vi "SetRemoteControl.vi"(0 "reference in":refnum<class "Button.lvclass">, 7 "RemoteControl":refnum<class "RemoteControl.lvclass">, 11 "Error In":errorcluster) -> (4 "reference out":refnum<class "Button.lvclass">, 15 "Error Out":errorcluster)   [LabVIEW 2024, in "Button.lvclass"]
uses:
  Button.lvclass
  RemoteControl_class/RemoteControl.lvclass
  Button.lvclass/Button.ctl
panel:
  # "Connector Pane"
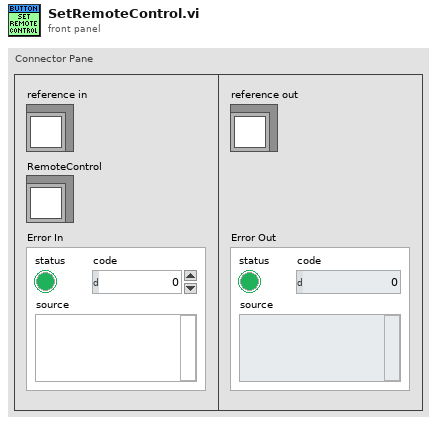
[diagram p1: front panel]
types:
  T1 = typedef "Button.lvclass/ObjectAttributes.ctl" = cluster{"RemoteControl":refnum<class "RemoteControl.lvclass">}
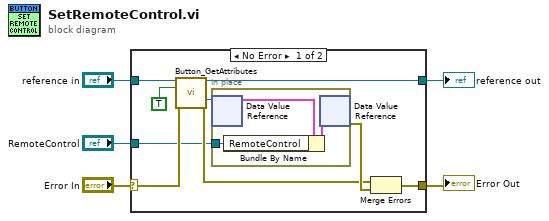
[diagram p0: block diagram]
diagram:
  n1 = case shown="No Error" "Error In" {
    selector: "Error In" -> [w12 w19]
    tunnel: [w7 w19] -> w4
    tunnel: [w13 w18] -> w2
    tunnel: "reference in" -> [w14 w18]
    tunnel: "RemoteControl" -> [w6 _]
    frame No Error {
      n2 = call "Button_GetAttributes.vi"("reference in"=w14, "OnlyGetDvrReference(False)"=TRUE, "Error In"=w12) -> ("reference out"=w13:refnum<class "Button.lvclass">, "DataRef"=w9:refnum<data-value>, "Error Out"=w8:errorcluster)  [unwired: 9 in, 1 out]
      n3 = in-place {
        in-place-border: w6 -> [w17]
        n4 = in-place-dvr #1(w9) -> (w16:T1)  [unwired: 1 out]
        n5 = Bundle By Name(cluster=w16, "RemoteControl"=w17) -> (w15:T1)
        n6 = in-place-dvr #1(w15) -> (w10:errorcluster)  [unwired: 1 out]
      }
      n7 = Merge Errors(w8, w10) -> (w7:errorcluster)
    }
    frame Error {
    }
  }
  "Error Out" <- w4
  "reference out" <- w2
